vi "UART Read.vi"(8 "error in (no error)":errorcluster, 11 "Read Length Limit":i32) -> (0 "error out":errorcluster, 2 "String Length":i32, 3 "String":string)   [LabVIEW 2011]
uses:
  Libraries/uart_library.dll
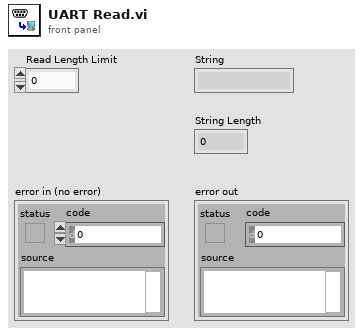
[diagram p1: front panel]
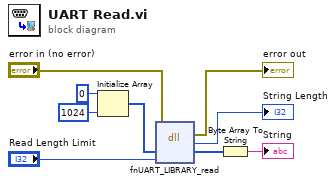
[diagram p0: block diagram]
diagram:
  n1 = Initialize Array(u8 0 ("element"), 1024 ("dimension size")) -> (w3:u8[])
  n2 = dll-call lib="E:/users/tba/work_project/FW102/trunk/LabVIEW/Libraries/uart_library.dll" fn="fnUART_LIBRARY_read"(error in="error in (no error)", "Return String"=w3, "Limit"="Read Length Limit") -> (error out=→"error out":errorcluster, "Return String Size"=→"String Length":i32, "Return String"=w2:u8[])  [unwired: 3 in, 1 out]
  n3 = Byte Array To String(unsigned byte array=w2) -> (string=→"String":string)
